vi "NewGame.vi"(8 "error in (no error)":errorcluster, 10 "Engine in":refnum<class "Engine.lvclass">, 11 "BounceDemoType (ChildObject)":refnum<class "BounceDemo.lvclass">) -> (0 "error out":errorcluster, 2 "Engine out":refnum<class "Engine.lvclass">, 3 "BounceDemo out":refnum<class "BounceDemo.lvclass">)   [LabVIEW 2019, in "RT_Game.lvlib" / "BounceDemo.lvclass"]
uses:
  BounceDemo.lvclass
  C:/Users/FreshBob/Dropbox/VIs/myRIO_GameConsole/RT/RT_Game/Game/Game.lvclass
  Engine/Engine.lvclass
  Game/Game.lvclass/Game.ctl
  BounceDemo.lvclass/BounceDemo.ctl
  Game/Write HasHighscore_.vi
  Game/Write HasMenu_.vi
  Bouncer/Bouncer.lvclass
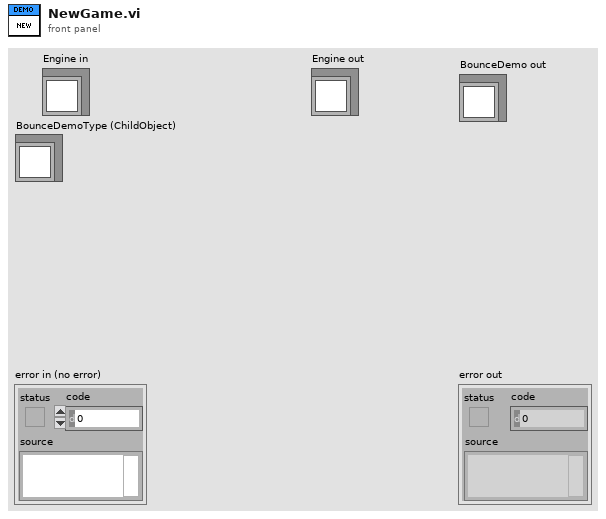
[diagram p1: front panel]
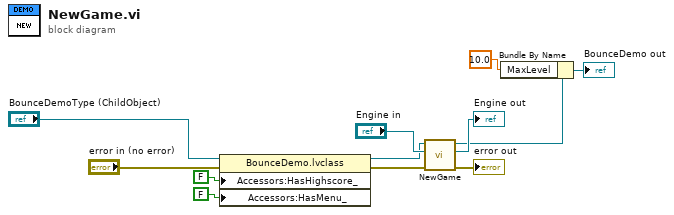
[diagram p0: block diagram]
diagram:
  n1 = property class="BounceDemo.lvclass"(reference="BounceDemoType (ChildObject)", error in="error in (no error)", "Accessors:HasHighscore_"=FALSE ("HasHighscore_"), "Accessors:HasMenu_"=FALSE ("HasMenu_")) -> (reference out=w5:refnum<class "BounceDemo.lvclass">, error out=w7:errorcluster)
  n2 = call-parent "NewGame.vi"("error in (no error)"=w7, "Engine in"="Engine in", "BouncerType (ChildObject)"=w5) -> ("error out"=→"error out":errorcluster, "Engine out"=→"Engine out":refnum<class "Engine.lvclass">, "Bouncer out"=w10:refnum<class "BounceDemo.lvclass">)  [unwired: 6 in]
  n3 = Bundle By Name(cluster=w10, "MaxLevel"=10.0 ("Duration")) -> (→"BounceDemo out":refnum<class "BounceDemo.lvclass">)
